vi "readArmEncoders.vi"() -> ()   [LabVIEW 2015]
panel:
  out "Encoder Output 3":i32
  in  "stop 2":bool
  in  "stop":bool
  out "Encoder Output 2":i32
  out "Encoder Output":i32
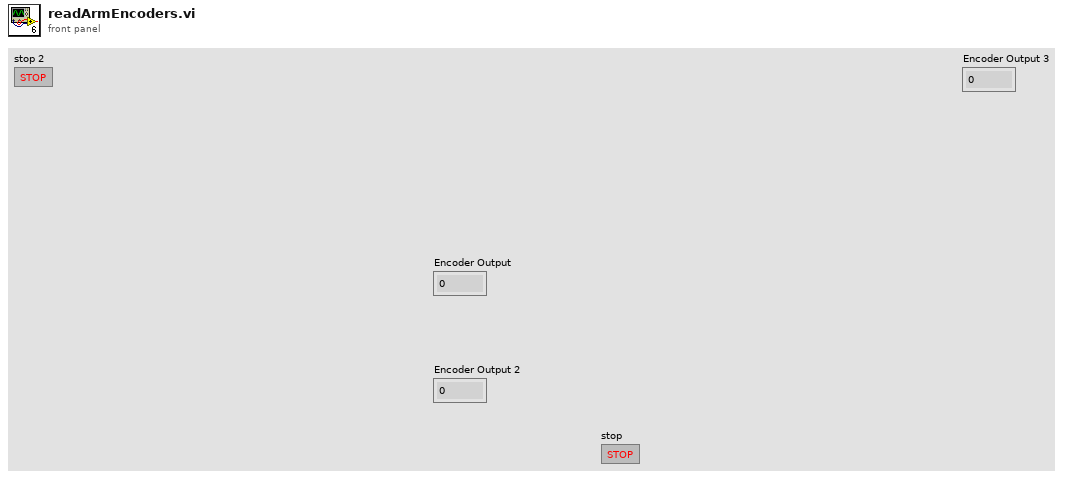
[diagram p1: front panel]
types:
  T1 = enum16{"shoulder", "elbow", "wrist", "base", "gripper"}
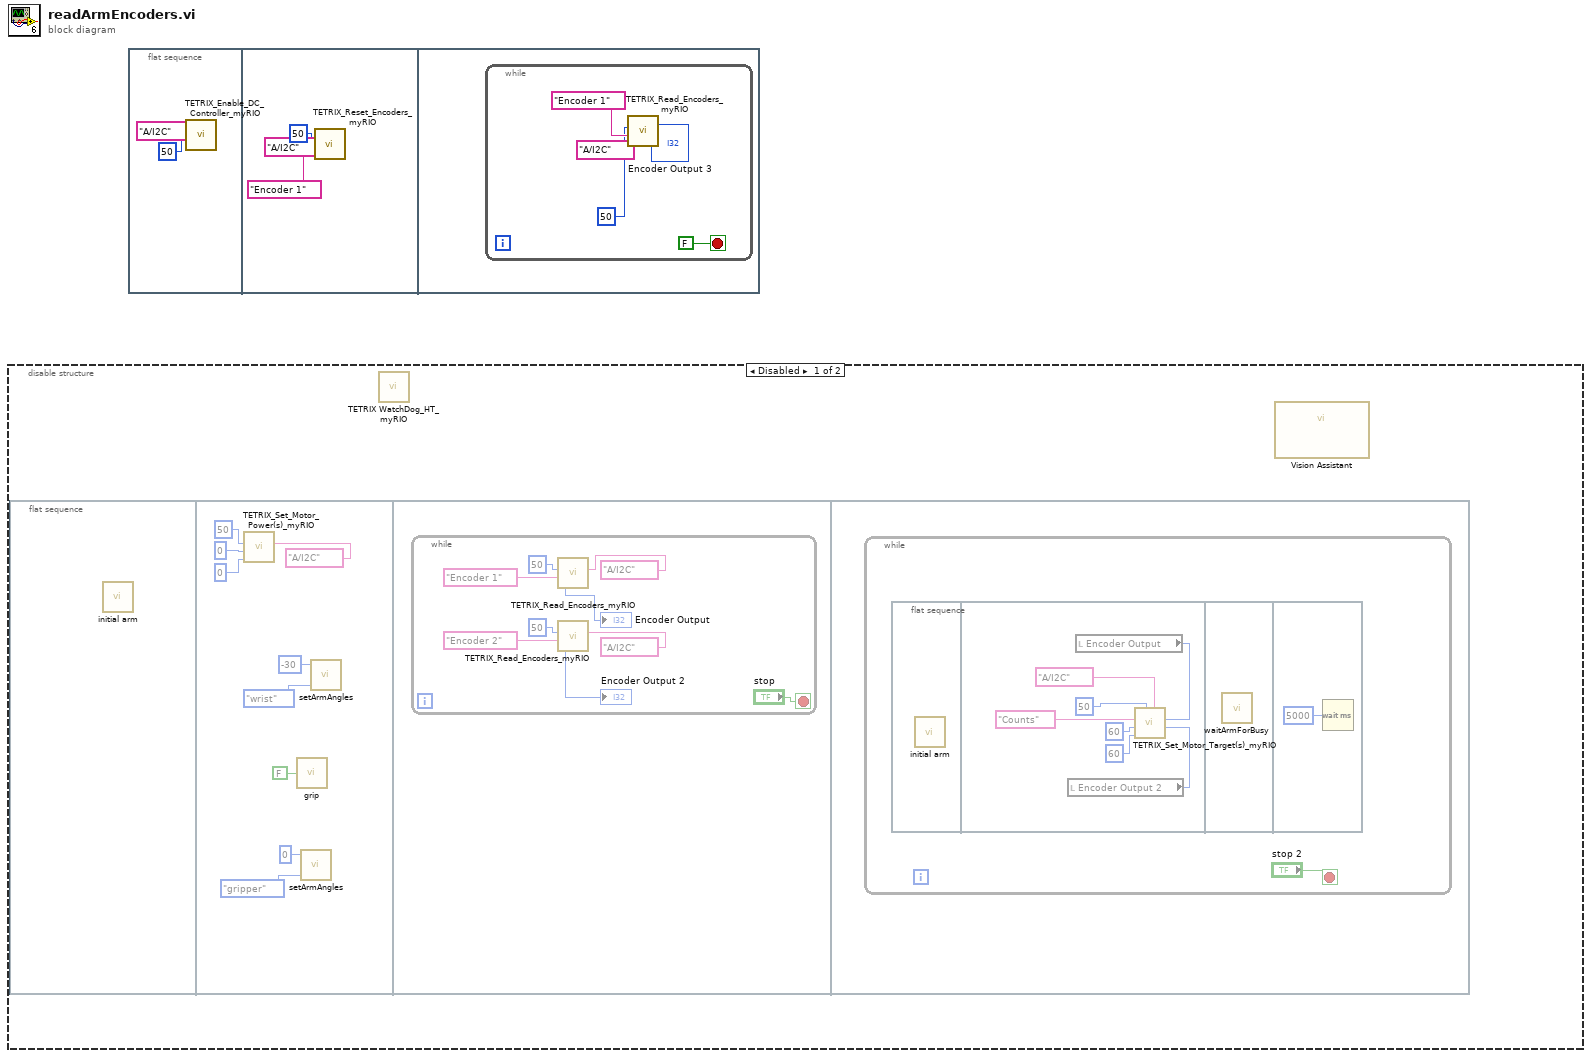
[diagram p0: block diagram]
diagram:
  n1 = disable-structure shown="Disabled" {
    frame Disabled {
      n2 = flat-sequence {
        frame #0 {
          n3 = call "initial arm.vi"() -> ()  [unwired: 12 in]
        }
        frame #1 {
          n4 = call <vilib>:"TETRIX_Set_Motor_Power(s)_myRIO.vi"("myRIO MXP Port A/B"=tag "A/I2C", "Motor 2 Power (-100 to 100)  0 = Coast Stop  125 = Brake Stop"=i8 0, "Motor 1 Power (-100 to 100)  0 = Coast Stop  125 = Brake Stop"=i8 0, "Controller ID#  (I2C Address)"=u8 50) -> ()  [unwired: 3 in, 1 out]
          n5 = call "grip.vi"("grip"=FALSE) -> ()
          n6 = call "setArmAngles.vi"("Enum"=T1."gripper", "angle"=0) -> ()  [unwired: 2 in]
          n7 = call "setArmAngles.vi"("Enum"=T1."wrist", "angle"=-30) -> ()  [unwired: 2 in]
        }
        frame #2 {
          n8 = while {
            stop <- "stop" stop-if-true
            n9 = call <vilib>:"TETRIX_Read_Encoders_myRIO.vi"("myRIO MXP Port A/B"=tag "A/I2C", "Select Encoder"="Encoder 1", "Controller ID#  (I2C Address)"=u8 50) -> ("Encoder Output"=→"Encoder Output":i32)  [unwired: 3 in, 1 out]
            n10 = call <vilib>:"TETRIX_Read_Encoders_myRIO.vi"("myRIO MXP Port A/B"=tag "A/I2C", "Select Encoder"="Encoder 2", "Controller ID#  (I2C Address)"=u8 50) -> ("Encoder Output"=→"Encoder Output 2":i32)  [unwired: 3 in, 1 out]
          }
        }
        frame #3 {
          n11 = while {
            stop <- "stop 2" stop-if-true
            n12 = flat-sequence {
              frame #0 {
                n13 = call "initial arm.vi"() -> ()  [unwired: 12 in]
              }
              frame #1 {
                n14 = local read "Encoder Output 2"() -> (w20:i32)
                n15 = local read "Encoder Output"() -> (w21:i32)
                n16 = call <vilib>:"TETRIX_Set_Motor_Target(s)_myRIO.vi"("Motor 2 Encoder Target"=w20, "Motor 1 Encoder Target"=w21, "myRIO MXP Port A/B"=tag "A/I2C", "Controller ID#  (I2C Address)"=u8 50, "Motor 2 Constant Speed (Degrees per Second)"=i16 60, "Motor 1 Contant Speed (Degrees per Second)"=i16 60, "Encoder Units"="Counts") -> ()  [unwired: 2 in, 1 out]
              }
              frame #2 {
                n17 = call "waitArmForBusy.vi"() -> ()  [unwired: 12 in]
              }
              frame #3 {
                n18 = Wait (ms)(milliseconds to wait=u32 5000) -> ()  [unwired: 1 out]
              }
            }
          }
        }
      }
      n19 = call <vilib>:"TETRIX WatchDog_HT_myRIO.vi"() -> ()  [unwired: 3 in, 1 out]
      n20 = call "Vision Assistant"() -> ()  [unwired: 12 in]
    }
    frame Enabled {
    }
  }
  n21 = flat-sequence {
    frame #0 {
      n22 = call <vilib>:"TETRIX_Enable_DC_Controller_myRIO.vi"("myRIO MXP Port A/B"=tag "A/I2C", "Controller ID#  (I2C Address)"=u8 50) -> ()  [unwired: 5 in, 1 out]
    }
    frame #1 {
      n23 = call <vilib>:"TETRIX_Reset_Encoders_myRIO.vi"("myRIO MXP Port A/B"=tag "A/I2C", "Select Encoder"="Encoder 1", "Controller ID#  (I2C Address)"=u8 50) -> ()  [unwired: 4 in, 1 out]
    }
    frame #2 {
      n24 = while {
        stop <- FALSE stop-if-true
        n25 = call <vilib>:"TETRIX_Read_Encoders_myRIO.vi"("myRIO MXP Port A/B"=tag "A/I2C", "Select Encoder"="Encoder 1", "Controller ID#  (I2C Address)"=u8 50) -> ("Encoder Output"=→"Encoder Output 3":i32)  [unwired: 3 in, 1 out]
      }
    }
  }
